vi "TDT-Set Target Val (DBL).vi"(0 "Data":T1={"TTankX"=refnum, "TDevAccX"=refnum, "LastTime"=0.0, "error"={"status"=FALSE, "code"=0, "source"=""}, "Block Name"="", "Circuit Tag"="", "Tank Name"="", "NumTicks"=0, "LastTick"=0.0, "Idle?"=FALSE, "Wait (ms)"=1000, "LastArtf"=0.0, "LastTosc"=0.0}, 7 "Target":string, 9 "Val":dbl, 11 "error in (no error)":errorcluster) -> (15 "error out":errorcluster)   [LabVIEW 2015]
uses:
  TDT Interface Data.ctl
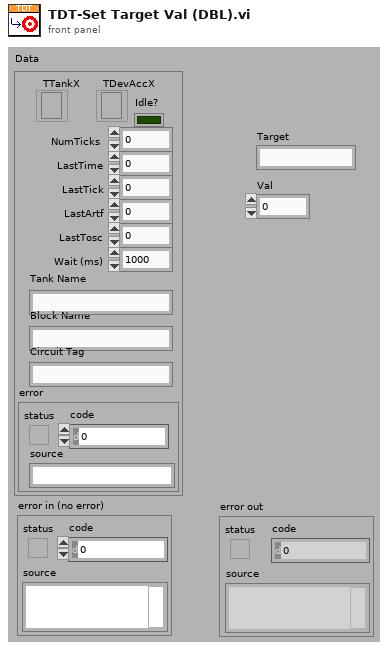
[diagram p1: front panel]
types:
  T1 = typedef "TDT Interface Data.ctl" = cluster{"TTankX":refnum<k7>, "TDevAccX":refnum<k7>, "LastTime":dbl, "error":errorcluster, "Block Name":string, "Circuit Tag":string, "Tank Name":string, "NumTicks":i32, "LastTick":dbl, "Idle?":bool, "Wait (ms)":u32, "LastArtf":dbl, "LastTosc":dbl}
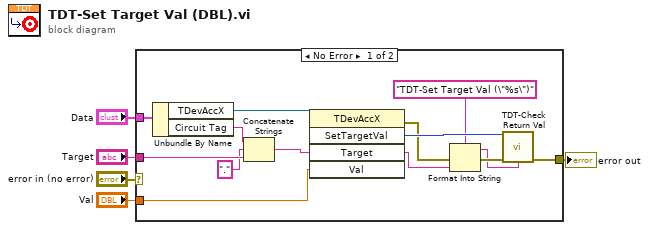
[diagram p0: block diagram]
diagram:
  n1 = case shown="No Error" "error in (no error)" {
    selector: "error in (no error)" -> [_ w20]
    tunnel: [w12 w20] -> w4
    tunnel: "Data" -> [w18 _]
    tunnel: "Target" -> [w16 _]
    tunnel: "Val" -> [w13 _]
    frame No Error {
      n2 = Unbundle By Name(w18) -> ("TDevAccX"=w19:refnum<k7>, "Circuit Tag"=w17:string)
      n3 = Concatenate Strings(w17, "." ("string"), w16) -> (w14:string)
      n4 = invoke class="TDevAccX" method="SetTargetVal"(reference=w19, "Target"=w14, "Val"=w13) -> (error out=w9:errorcluster, "SetTargetVal"=w11:i32, "Target"=w8:string)  [unwired: 2 in, 2 out]
      n5 = Format Into String(format string="TDT-Set Target Val (\"%s\")" ("source"), error in=w9, w8) -> (resulting string=w7:string, error out=w10:errorcluster)  [unwired: 1 in]
      n6 = call "TDT-Check Return Val.vi"("Return Val"=w11, "error in (no error)"=w10, "source"=w7) -> ("error out"=w12:errorcluster)  [unwired: 12 in]
    }
    frame Error {
    }
  }
  "error out" <- w4
